vi "INSTRUMENTORDERS.vi"(7 "错误输入（无错误）":errorcluster, 8 "关闭通道":u16(ring) items=["CH1", "CH2", "CH3", "CH4"], 9 "打开通道":u16(ring) items=["CH1", "CH2", "CH3", "CH4"], 10 "VISA资源名称":refnum<visa-resource-name>="DPO5054-C012667") -> (0 "错误输出":errorcluster, 2 "输出数组":dbl[](array[numeric]))   [LabVIEW 2014]
panel:
  out "ACRMS":dbl
  out "NegativeDutyCycle":dbl
  out "PositiveDutyCycle":dbl
  out "NegWidth":dbl
  out "PosWidth":dbl
  out "FallTime":dbl
  out "RISETIME":dbl
  out "FREQ":dbl
  out "PERIOD":dbl
  out "PK2PK":dbl
  out "MIN":dbl
  out "MAX":dbl
  out "RMS":dbl
  out "AMP":dbl
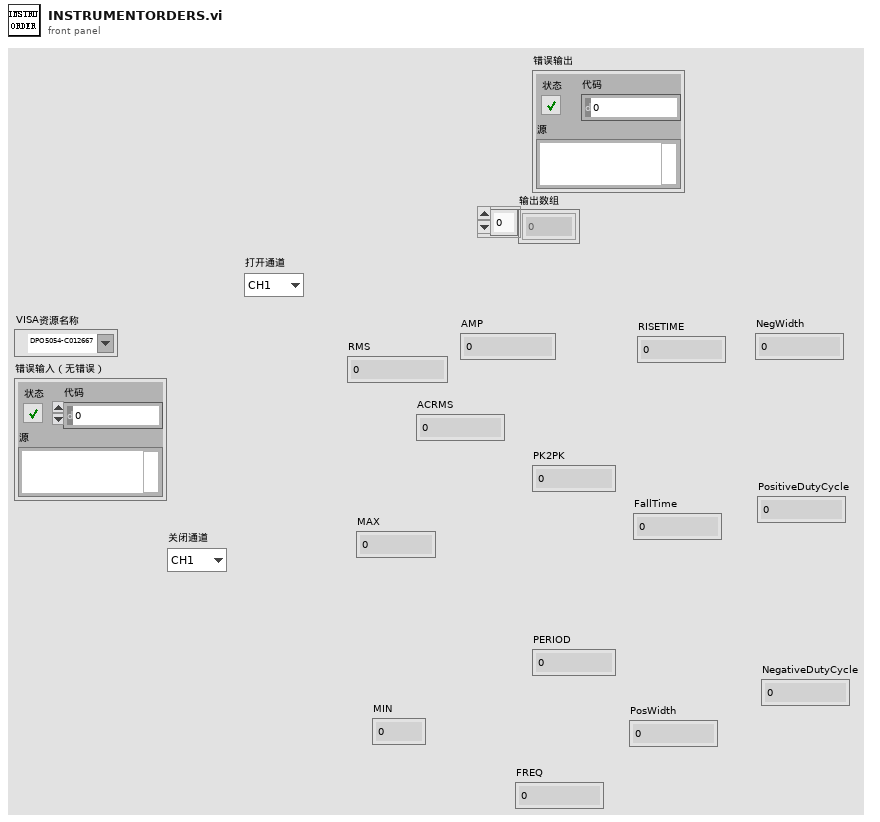
[diagram p1: front panel]
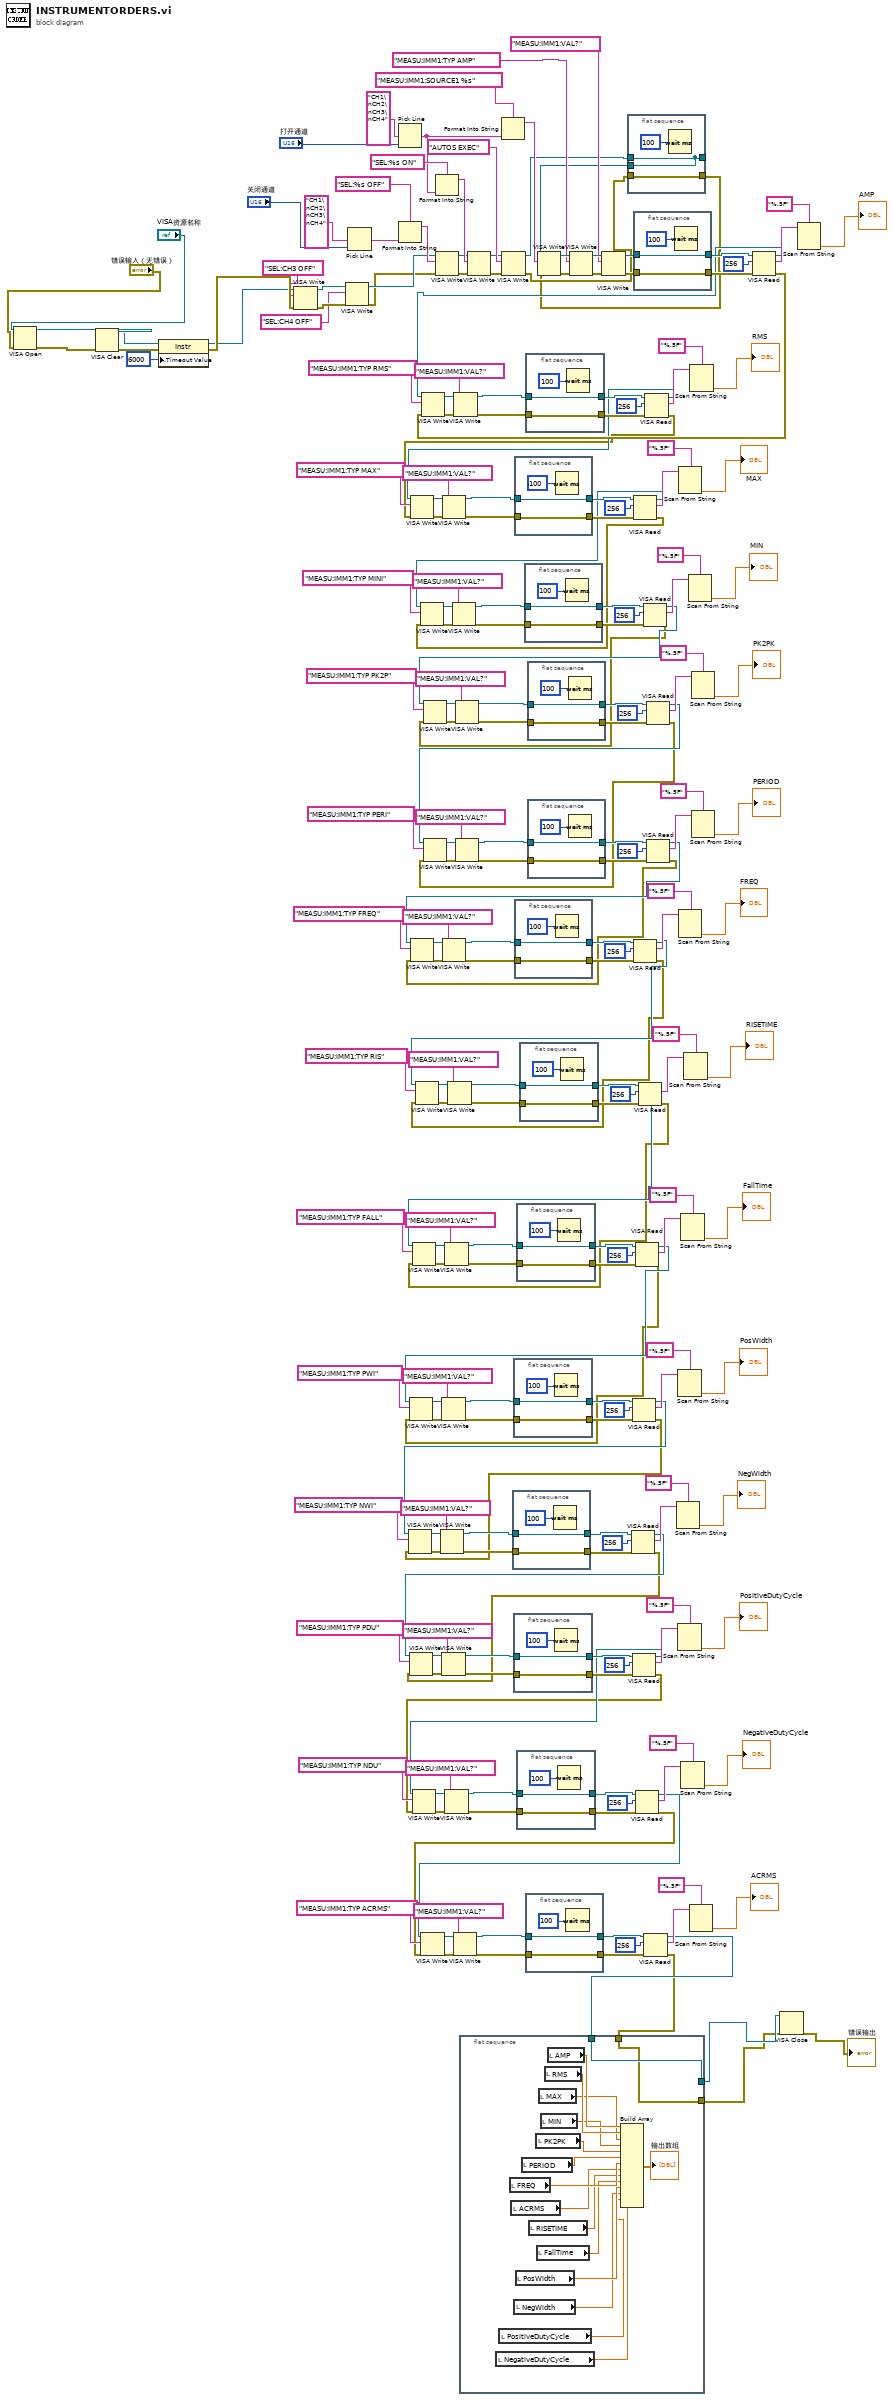
[diagram p0: block diagram]
diagram:
  n1 = VISA Open(error in (no error)="错误输入（无错误）", VISA resource name="VISA资源名称") -> (VISA resource name=w17:refnum<visa-resource-name>, error out=w16:errorcluster)  [unwired: 3 in]
  n2 = VISA Clear(VISA resource name=w17, error in (no error)=w16) -> (VISA resource name out=w15:refnum<visa-resource-name>, error out=w14:errorcluster)
  n3 = property class="Instr"(reference=w15, error in=w14, "General Settings:Timeout Value"=u32 6000) -> (reference out=w7:refnum<visa-resource-name>, error out=w8:errorcluster)
  n4 = VISA Write(VISA resource name=w7, write buffer="SEL:CH3 OFF" ("格式字符串"), error in (no error)=w8) -> (VISA resource name out=w5:refnum<visa-resource-name>, error out=w4:errorcluster)  [unwired: 1 out]
  n5 = VISA Write(VISA resource name=w5, write buffer="SEL:CH4 OFF" ("格式字符串"), error in (no error)=w4) -> (VISA resource name out=w2:refnum<visa-resource-name>, error out=w1:errorcluster)  [unwired: 1 out]
  n6 = Pick Line(multi-line string="CH1\nCH2\nCH3\nCH4" ("多行字符串"), line index="关闭通道") -> (output string=w217:string)  [unwired: 1 in]
  n7 = Pick Line(multi-line string="CH1\nCH2\nCH3\nCH4" ("多行字符串"), line index="打开通道") -> (output string=w222:string)  [unwired: 1 in]
  n8 = Format Into String(format string="SEL:%s OFF" ("格式字符串"), w217) -> (resulting string=w213:string)  [unwired: 2 in, 1 out]
  n9 = Format Into String(format string="SEL:%s ON" ("格式字符串"), w222) -> (resulting string=w221:string)  [unwired: 2 in, 1 out]
  n10 = VISA Write(VISA resource name=w2, write buffer=w213, error in (no error)=w1) -> (VISA resource name out=w212:refnum<visa-resource-name>, error out=w211:errorcluster)  [unwired: 1 out]
  n11 = flat-sequence {
    tunnel: w20 -> [w239]
    tunnel: [w239] -> w11
    tunnel: w19 -> [w238]
    tunnel: [w238] -> w10
    frame #0 {
      n12 = local read "NegativeDutyCycle"() -> (w241:dbl)
      n13 = local read "PositiveDutyCycle"() -> (w242:dbl)
      n14 = local read "FREQ"() -> (w248:dbl)
      n15 = local read "ACRMS"() -> (w247:dbl)
      n16 = local read "NegWidth"() -> (w243:dbl)
      n17 = local read "PosWidth"() -> (w244:dbl)
      n18 = local read "PERIOD"() -> (w249:dbl)
      n19 = local read "RISETIME"() -> (w246:dbl)
      n20 = local read "PK2PK"() -> (w250:dbl)
      n21 = local read "FallTime"() -> (w245:dbl)
      n22 = local read "MAX"() -> (w252:dbl)
      n23 = local read "MIN"() -> (w251:dbl)
      n24 = local read "RMS"() -> (w253:dbl)
      n25 = local read "AMP"() -> (w254:dbl)
      n26 = Build Array(w254, w253, w252, w251, w250, w249, w248, w247, w246, w245, w244, w243, w242, w241) -> (→"输出数组":dbl[])
    }
  }
  n27 = VISA Write(VISA resource name=w212, write buffer=w221, error in (no error)=w211) -> (VISA resource name out=w219:refnum<visa-resource-name>, error out=w218:errorcluster)  [unwired: 1 out]
  n28 = Format Into String(format string="MEASU:IMM1:SOURCE1 %s" ("格式字符串"), w222) -> (resulting string=w235:string)  [unwired: 2 in, 1 out]
  n29 = VISA Write(VISA resource name=w219, write buffer="AUTOS EXEC" ("写入缓冲区"), error in (no error)=w218) -> (VISA resource name out=w122:refnum<visa-resource-name>, error out=w121:errorcluster)  [unwired: 1 out]
  n30 = flat-sequence {
    tunnel: w81 -> [w256]
    tunnel: [w256] -> w79
    tunnel: w82 -> [w255]
    tunnel: [w255] -> w78
    frame #0 {
      n31 = Wait (ms)(milliseconds to wait=u32 100 ("等待时间（毫秒）")) -> ()  [unwired: 1 out]
    }
  }
  n32 = flat-sequence {
    tunnel: w84 -> [w259]
    tunnel: [w259] -> w86
    tunnel: w83 -> [w258]
    tunnel: [w258] -> w87
    frame #0 {
      n33 = Wait (ms)(milliseconds to wait=u32 100 ("等待时间（毫秒）")) -> ()  [unwired: 1 out]
    }
  }
  n34 = flat-sequence {
    tunnel: w60 -> [w262]
    tunnel: [w262] -> w62
    tunnel: w59 -> [w261]
    tunnel: [w261] -> w63
    frame #0 {
      n35 = Wait (ms)(milliseconds to wait=u32 100 ("等待时间（毫秒）")) -> ()  [unwired: 1 out]
    }
  }
  n36 = flat-sequence {
    tunnel: w193 -> [w265]
    tunnel: [w265] -> w191
    tunnel: w194 -> [w264]
    tunnel: [w264] -> w190
    frame #0 {
      n37 = Wait (ms)(milliseconds to wait=u32 100 ("等待时间（毫秒）")) -> ()  [unwired: 1 out]
    }
  }
  n38 = flat-sequence {
    tunnel: w145 -> [w268]
    tunnel: [w268] -> w143
    tunnel: w146 -> [w267]
    tunnel: [w267] -> w142
    frame #0 {
      n39 = Wait (ms)(milliseconds to wait=u32 100 ("等待时间（毫秒）")) -> ()  [unwired: 1 out]
    }
  }
  n40 = flat-sequence {
    tunnel: w105 -> [w271]
    tunnel: [w271] -> w103
    tunnel: w106 -> [w270]
    tunnel: [w270] -> w102
    frame #0 {
      n41 = Wait (ms)(milliseconds to wait=u32 100 ("等待时间（毫秒）")) -> ()  [unwired: 1 out]
    }
  }
  n42 = flat-sequence {
    tunnel: w57 -> [w274]
    tunnel: [w274] -> w55
    tunnel: w58 -> [w273]
    tunnel: [w273] -> w54
    frame #0 {
      n43 = Wait (ms)(milliseconds to wait=u32 100 ("等待时间（毫秒）")) -> ()  [unwired: 1 out]
    }
  }
  n44 = flat-sequence {
    tunnel: w108 -> [w277]
    tunnel: [w277] -> w110
    tunnel: w107 -> [w276]
    tunnel: [w276] -> w111
    frame #0 {
      n45 = Wait (ms)(milliseconds to wait=u32 100 ("等待时间（毫秒）")) -> ()  [unwired: 1 out]
    }
  }
  n46 = flat-sequence {
    tunnel: w172 -> [w280]
    tunnel: [w280] -> w174
    tunnel: w171 -> [w279]
    tunnel: [w279] -> w175
    frame #0 {
      n47 = Wait (ms)(milliseconds to wait=u32 100 ("等待时间（毫秒）")) -> ()  [unwired: 1 out]
    }
  }
  n48 = flat-sequence {
    tunnel: w24 -> [w283]
    tunnel: [w283] -> w26
    tunnel: w23 -> [w282]
    tunnel: [w282] -> w27
    frame #0 {
      n49 = Wait (ms)(milliseconds to wait=u32 100 ("等待时间（毫秒）")) -> ()  [unwired: 1 out]
    }
  }
  n50 = flat-sequence {
    tunnel: w196 -> [w286]
    tunnel: [w286] -> w198
    tunnel: w195 -> [w285]
    tunnel: [w285] -> w199
    frame #0 {
      n51 = Wait (ms)(milliseconds to wait=u32 100 ("等待时间（毫秒）")) -> ()  [unwired: 1 out]
    }
  }
  n52 = flat-sequence {
    tunnel: w169 -> [w289]
    tunnel: [w289] -> w167
    tunnel: w170 -> [w288]
    tunnel: [w288] -> w166
    frame #0 {
      n53 = Wait (ms)(milliseconds to wait=u32 100 ("等待时间（毫秒）")) -> ()  [unwired: 1 out]
    }
  }
  n54 = flat-sequence {
    tunnel: w148 -> [w292]
    tunnel: [w292] -> w150
    tunnel: w147 -> [w291]
    tunnel: [w291] -> w151
    frame #0 {
      n55 = Wait (ms)(milliseconds to wait=u32 100 ("等待时间（毫秒）")) -> ()  [unwired: 1 out]
    }
  }
  n56 = VISA Write(VISA resource name=w120, write buffer=w235, error in (no error)=w119) -> (VISA resource name out=w232:refnum<visa-resource-name>, error out=w231:errorcluster)  [unwired: 1 out]
  n57 = VISA Write(VISA resource name=w232, write buffer="MEASU:IMM1:TYP AMP" ("写入缓冲区"), error in (no error)=w231) -> (VISA resource name out=w228:refnum<visa-resource-name>, error out=w227:errorcluster)  [unwired: 1 out]
  n58 = VISA Write(VISA resource name=w228, write buffer="MEASU:IMM1:VAL?" ("写入缓冲区"), error in (no error)=w227) -> (VISA resource name out=w225:refnum<visa-resource-name>, error out=w224:errorcluster)  [unwired: 1 out]
  n59 = flat-sequence {
    tunnel: w122 -> [w294]
    tunnel: [w294] -> _
    tunnel: w121 -> [w295]
    tunnel: [w295] -> w119
    tunnel: [w294] -> w120
    frame #0 {
      n60 = Wait (ms)(milliseconds to wait=u32 100 ("等待时间（毫秒）")) -> ()  [unwired: 1 out]
    }
  }
  n61 = VISA Read(VISA resource name=w79, byte count=u32 256 ("字节总数"), error in (no error)=w78) -> (VISA resource name out=w38:refnum<visa-resource-name>, read buffer=w77:string, error out=w37:errorcluster)  [unwired: 1 out]
  n62 = VISA Write(VISA resource name=w38, write buffer="MEASU:IMM1:TYP PDU" ("写入缓冲区"), error in (no error)=w37) -> (VISA resource name out=w68:refnum<visa-resource-name>, error out=w69:errorcluster)  [unwired: 1 out]
  n63 = VISA Write(VISA resource name=w68, write buffer="MEASU:IMM1:VAL?" ("写入缓冲区"), error in (no error)=w69) -> (VISA resource name out=w60:refnum<visa-resource-name>, error out=w59:errorcluster)  [unwired: 1 out]
  n64 = VISA Read(VISA resource name=w86, byte count=u32 256 ("字节总数"), error in (no error)=w87) -> (VISA resource name out=w40:refnum<visa-resource-name>, read buffer=w88:string, error out=w39:errorcluster)  [unwired: 1 out]
  n65 = VISA Write(VISA resource name=w40, write buffer="MEASU:IMM1:TYP NWI" ("写入缓冲区"), error in (no error)=w39) -> (VISA resource name out=w73:refnum<visa-resource-name>, error out=w72:errorcluster)  [unwired: 1 out]
  n66 = VISA Write(VISA resource name=w73, write buffer="MEASU:IMM1:VAL?" ("写入缓冲区"), error in (no error)=w72) -> (VISA resource name out=w81:refnum<visa-resource-name>, error out=w82:errorcluster)  [unwired: 1 out]
  n67 = VISA Read(VISA resource name=w62, byte count=u32 256 ("字节总数"), error in (no error)=w63) -> (VISA resource name out=w36:refnum<visa-resource-name>, read buffer=w64:string, error out=w35:errorcluster)  [unwired: 1 out]
  n68 = VISA Write(VISA resource name=w36, write buffer="MEASU:IMM1:TYP NDU" ("写入缓冲区"), error in (no error)=w35) -> (VISA resource name out=w49:refnum<visa-resource-name>, error out=w48:errorcluster)  [unwired: 1 out]
  n69 = VISA Write(VISA resource name=w49, write buffer="MEASU:IMM1:VAL?" ("写入缓冲区"), error in (no error)=w48) -> (VISA resource name out=w57:refnum<visa-resource-name>, error out=w58:errorcluster)  [unwired: 1 out]
  n70 = flat-sequence {
    tunnel: w225 -> [w298]
    tunnel: [w298] -> w230
    tunnel: w224 -> [w297]
    tunnel: [w297] -> w229
    frame #0 {
      n71 = Wait (ms)(milliseconds to wait=u32 100 ("等待时间（毫秒）")) -> ()  [unwired: 1 out]
    }
  }
  n72 = VISA Read(VISA resource name=w191, byte count=u32 256 ("字节总数"), error in (no error)=w190) -> (VISA resource name out=w130:refnum<visa-resource-name>, read buffer=w189:string, error out=w129:errorcluster)  [unwired: 1 out]
  n73 = VISA Write(VISA resource name=w130, write buffer="MEASU:IMM1:TYP MINI" ("写入缓冲区"), error in (no error)=w129) -> (VISA resource name out=w180:refnum<visa-resource-name>, error out=w181:errorcluster)  [unwired: 1 out]
  n74 = VISA Write(VISA resource name=w180, write buffer="MEASU:IMM1:VAL?" ("写入缓冲区"), error in (no error)=w181) -> (VISA resource name out=w172:refnum<visa-resource-name>, error out=w171:errorcluster)  [unwired: 1 out]
  n75 = VISA Read(VISA resource name=w143, byte count=u32 256 ("字节总数"), error in (no error)=w142) -> (VISA resource name out=w46:refnum<visa-resource-name>, read buffer=w141:string, error out=w45:errorcluster)  [unwired: 1 out]
  n76 = VISA Write(VISA resource name=w46, write buffer="MEASU:IMM1:TYP RIS" ("写入缓冲区"), error in (no error)=w45) -> (VISA resource name out=w116:refnum<visa-resource-name>, error out=w117:errorcluster)  [unwired: 1 out]
  n77 = VISA Write(VISA resource name=w116, write buffer="MEASU:IMM1:VAL?" ("写入缓冲区"), error in (no error)=w117) -> (VISA resource name out=w108:refnum<visa-resource-name>, error out=w107:errorcluster)  [unwired: 1 out]
  n78 = VISA Read(VISA resource name=w103, byte count=u32 256 ("字节总数"), error in (no error)=w102) -> (VISA resource name out=w42:refnum<visa-resource-name>, read buffer=w101:string, error out=w41:errorcluster)  [unwired: 1 out]
  n79 = VISA Write(VISA resource name=w42, write buffer="MEASU:IMM1:TYP PWI" ("写入缓冲区"), error in (no error)=w41) -> (VISA resource name out=w92:refnum<visa-resource-name>, error out=w93:errorcluster)  [unwired: 1 out]
  n80 = VISA Write(VISA resource name=w92, write buffer="MEASU:IMM1:VAL?" ("写入缓冲区"), error in (no error)=w93) -> (VISA resource name out=w84:refnum<visa-resource-name>, error out=w83:errorcluster)  [unwired: 1 out]
  n81 = VISA Read(VISA resource name=w55, byte count=u32 256 ("字节总数"), error in (no error)=w54) -> (VISA resource name out=w22:refnum<visa-resource-name>, read buffer=w53:string, error out=w21:errorcluster)  [unwired: 1 out]
  n82 = VISA Write(VISA resource name=w22, write buffer="MEASU:IMM1:TYP ACRMS" ("写入缓冲区"), error in (no error)=w21) -> (VISA resource name out=w32:refnum<visa-resource-name>, error out=w33:errorcluster)  [unwired: 1 out]
  n83 = VISA Write(VISA resource name=w32, write buffer="MEASU:IMM1:VAL?" ("写入缓冲区"), error in (no error)=w33) -> (VISA resource name out=w24:refnum<visa-resource-name>, error out=w23:errorcluster)  [unwired: 1 out]
  n84 = VISA Read(VISA resource name=w110, byte count=u32 256 ("字节总数"), error in (no error)=w111) -> (VISA resource name out=w44:refnum<visa-resource-name>, read buffer=w112:string, error out=w43:errorcluster)  [unwired: 1 out]
  n85 = VISA Write(VISA resource name=w44, write buffer="MEASU:IMM1:TYP FALL" ("写入缓冲区"), error in (no error)=w43) -> (VISA resource name out=w97:refnum<visa-resource-name>, error out=w96:errorcluster)  [unwired: 1 out]
  n86 = VISA Write(VISA resource name=w97, write buffer="MEASU:IMM1:VAL?" ("写入缓冲区"), error in (no error)=w96) -> (VISA resource name out=w105:refnum<visa-resource-name>, error out=w106:errorcluster)  [unwired: 1 out]
  n87 = VISA Read(VISA resource name=w174, byte count=u32 256 ("字节总数"), error in (no error)=w175) -> (VISA resource name out=w128:refnum<visa-resource-name>, read buffer=w176:string, error out=w127:errorcluster)  [unwired: 1 out]
  n88 = VISA Write(VISA resource name=w128, write buffer="MEASU:IMM1:TYP PK2P" ("写入缓冲区"), error in (no error)=w127) -> (VISA resource name out=w161:refnum<visa-resource-name>, error out=w160:errorcluster)  [unwired: 1 out]
  n89 = VISA Write(VISA resource name=w161, write buffer="MEASU:IMM1:VAL?" ("写入缓冲区"), error in (no error)=w160) -> (VISA resource name out=w169:refnum<visa-resource-name>, error out=w170:errorcluster)  [unwired: 1 out]
  n90 = VISA Read(VISA resource name=w26, byte count=u32 256 ("字节总数"), error in (no error)=w27) -> (VISA resource name out=w20:refnum<visa-resource-name>, read buffer=w28:string, error out=w19:errorcluster)  [unwired: 1 out]
  n91 = VISA Read(VISA resource name=w198, byte count=u32 256 ("字节总数"), error in (no error)=w199) -> (VISA resource name out=w132:refnum<visa-resource-name>, read buffer=w200:string, error out=w131:errorcluster)  [unwired: 1 out]
  n92 = VISA Write(VISA resource name=w132, write buffer="MEASU:IMM1:TYP MAX" ("写入缓冲区"), error in (no error)=w131) -> (VISA resource name out=w185:refnum<visa-resource-name>, error out=w184:errorcluster)  [unwired: 1 out]
  n93 = VISA Write(VISA resource name=w185, write buffer="MEASU:IMM1:VAL?" ("写入缓冲区"), error in (no error)=w184) -> (VISA resource name out=w193:refnum<visa-resource-name>, error out=w194:errorcluster)  [unwired: 1 out]
  n94 = VISA Read(VISA resource name=w167, byte count=u32 256 ("字节总数"), error in (no error)=w166) -> (VISA resource name out=w126:refnum<visa-resource-name>, read buffer=w165:string, error out=w125:errorcluster)  [unwired: 1 out]
  n95 = VISA Write(VISA resource name=w126, write buffer="MEASU:IMM1:TYP PERI" ("写入缓冲区"), error in (no error)=w125) -> (VISA resource name out=w156:refnum<visa-resource-name>, error out=w157:errorcluster)  [unwired: 1 out]
  n96 = VISA Write(VISA resource name=w156, write buffer="MEASU:IMM1:VAL?" ("写入缓冲区"), error in (no error)=w157) -> (VISA resource name out=w148:refnum<visa-resource-name>, error out=w147:errorcluster)  [unwired: 1 out]
  n97 = VISA Read(VISA resource name=w150, byte count=u32 256 ("字节总数"), error in (no error)=w151) -> (VISA resource name out=w124:refnum<visa-resource-name>, read buffer=w152:string, error out=w123:errorcluster)  [unwired: 1 out]
  n98 = VISA Write(VISA resource name=w124, write buffer="MEASU:IMM1:TYP FREQ" ("写入缓冲区"), error in (no error)=w123) -> (VISA resource name out=w137:refnum<visa-resource-name>, error out=w136:errorcluster)  [unwired: 1 out]
  n99 = VISA Write(VISA resource name=w137, write buffer="MEASU:IMM1:VAL?" ("写入缓冲区"), error in (no error)=w136) -> (VISA resource name out=w145:refnum<visa-resource-name>, error out=w146:errorcluster)  [unwired: 1 out]
  n100 = Scan From String(format string="%.5F" ("格式字符串"), input string=w77) -> (output 1=→"NegWidth":dbl)  [unwired: 3 in, 3 out]
  n101 = Scan From String(format string="%.5F" ("格式字符串"), input string=w88) -> (output 1=→"PosWidth":dbl)  [unwired: 3 in, 3 out]
  n102 = Scan From String(format string="%.5F" ("格式字符串"), input string=w64) -> (output 1=→"PositiveDutyCycle":dbl)  [unwired: 3 in, 3 out]
  n103 = Scan From String(format string="%.5F" ("格式字符串"), input string=w189) -> (output 1=→"MAX":dbl)  [unwired: 3 in, 3 out]
  n104 = Scan From String(format string="%.5F" ("格式字符串"), input string=w141) -> (output 1=→"FREQ":dbl)  [unwired: 3 in, 3 out]
  n105 = Scan From String(format string="%.5F" ("格式字符串"), input string=w101) -> (output 1=→"FallTime":dbl)  [unwired: 3 in, 3 out]
  n106 = Scan From String(format string="%.5F" ("格式字符串"), input string=w53) -> (output 1=→"NegativeDutyCycle":dbl)  [unwired: 3 in, 3 out]
  n107 = Scan From String(format string="%.5F" ("格式字符串"), input string=w112) -> (output 1=→"RISETIME":dbl)  [unwired: 3 in, 3 out]
  n108 = Scan From String(format string="%.5F" ("格式字符串"), input string=w176) -> (output 1=→"MIN":dbl)  [unwired: 3 in, 3 out]
  n109 = Scan From String(format string="%.5F" ("格式字符串"), input string=w28) -> (output 1=→"ACRMS":dbl)  [unwired: 3 in, 3 out]
  n110 = Scan From String(format string="%.5F" ("格式字符串"), input string=w200) -> (output 1=→"RMS":dbl)  [unwired: 3 in, 3 out]
  n111 = Scan From String(format string="%.5F" ("格式字符串"), input string=w165) -> (output 1=→"PK2PK":dbl)  [unwired: 3 in, 3 out]
  n112 = Scan From String(format string="%.5F" ("格式字符串"), input string=w152) -> (output 1=→"PERIOD":dbl)  [unwired: 3 in, 3 out]
  n113 = VISA Read(VISA resource name=w230, byte count=u32 256 ("字节总数"), error in (no error)=w229) -> (VISA resource name out=w134:refnum<visa-resource-name>, read buffer=w209:string, error out=w133:errorcluster)  [unwired: 1 out]
  n114 = VISA Write(VISA resource name=w134, write buffer="MEASU:IMM1:TYP RMS" ("写入缓冲区"), error in (no error)=w133) -> (VISA resource name out=w204:refnum<visa-resource-name>, error out=w205:errorcluster)  [unwired: 1 out]
  n115 = VISA Write(VISA resource name=w204, write buffer="MEASU:IMM1:VAL?" ("写入缓冲区"), error in (no error)=w205) -> (VISA resource name out=w196:refnum<visa-resource-name>, error out=w195:errorcluster)  [unwired: 1 out]
  n116 = VISA Close(VISA resource name=w11, error in (no error)=w10) -> (error out=→"错误输出":errorcluster)
  n117 = Scan From String(format string="%.5F" ("格式字符串"), input string=w209) -> (output 1=→"AMP":dbl)  [unwired: 3 in, 3 out]
